vi "gyro.vi"(0 "startspeed":dbl, 1 "left":dbl, 5 "kp- left":dbl, 7 "kp- right":dbl, 9 "kp+ left":dbl, 11 "kp+ right":dbl, 12 "right":dbl) -> ()   [LabVIEW 2016]
uses:
  <vilib>/Rock Robotics/WPI/Utilities/WPI_GetSetVariantRefNum.vi
panel:
  out "angle 2":dbl
  out "pi":dbl
  out "angle":dbl=360.0
  in  "Delay (s)":dbl
  in  "Feed time (s)":dbl=0.05
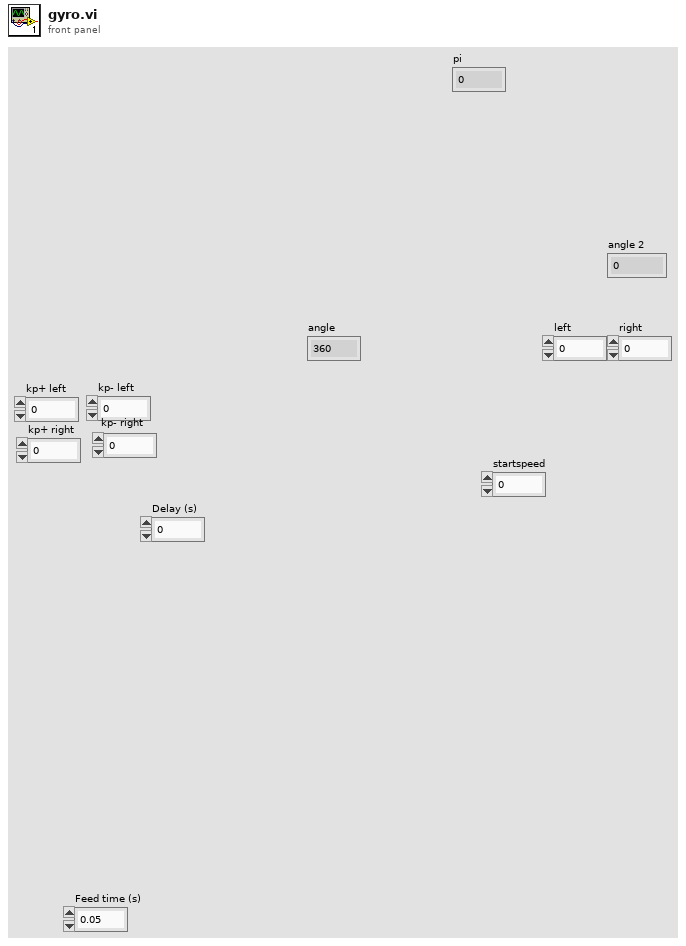
[diagram p1: front panel]
types:
  T1 = typedef "WPI_GyroDevRef.ctl" = cluster{"DevStatus":errorcluster, "Analog Channel":T2, "Offset":dbl, "Gain (VoltsPerDegree/Second)":dbl, "Gyro Type":enum16{"Analog", "XRS450"}, "Handle":i32, "SPI Bus":T3, "Device Found":bool, "Sample Rate":dbl, "Calibrate On Open":bool}
  T2 = typedef "FPGA_AIChannel.ctl" = enum8{"AI 0", "AI 1", "AI 2", "AI 3", "AI MXP 0", "AI MXP 1", "AI MXP 2", "AI MXP 3", "Invalid"}
  T3 = typedef "spi_bus.ctl" = enum16{"SPI On-Board, CS0", "SPI On-Board, CS1", "SPI On-Board, CS2", "SPI On-Board, CS3", "SPI MXP", "Invalid"}
  T4 = typedef "WPI_RobotDriveDevRef.ctl" = cluster{"DevStatus":errorcluster, "Motors[]":T5[], "Square Inputs":bool, "Max Output":dbl}
  T5 = typedef "WPI_MotorControlDeviceRef.ctl" = cluster{"DeviceStatus":errorcluster, "Type":T6, "PWM":cluster{"PWM Channel":T7, "DeadBand":T8}, "CAN":cluster{"Device Number":u8, "SetOutput VI Ref":variant, "GetOutput VI Ref":variant, "Enable VI Ref":variant, "Disable VI Ref":variant, "Data":variant}, "Invert":bool}
  T6 = typedef "WPI_MotorControlType.ctl" = enum16{"PWM", "CAN"}
  T7 = typedef "FPGA_DIOPWMChannel.ctl" = enum8{"PWM 0", "PWM 1", "PWM 2", "PWM 3", "PWM 4", "PWM 5", "PWM 6", "PWM 7", "PWM 8", "PWM 9", "PWM MXP 0", "PWM MXP 1", "PWM MXP 2", "PWM MXP 3", "PWM MXP 4", "PWM MXP 5", "PWM MXP 6", "PWM MXP 7", "PWM MXP 8", "PWM MXP 9", "Invalid"}
  T8 = typedef "WPI_PWMDeadband.ctl" = cluster{"Name":string, "maxPositivePwm":i32, "minPositivePwm":i32, "centerPwm":i32, "maxNegativePwm":i32, "minNegativePwm":i32, "angularRange":u16}
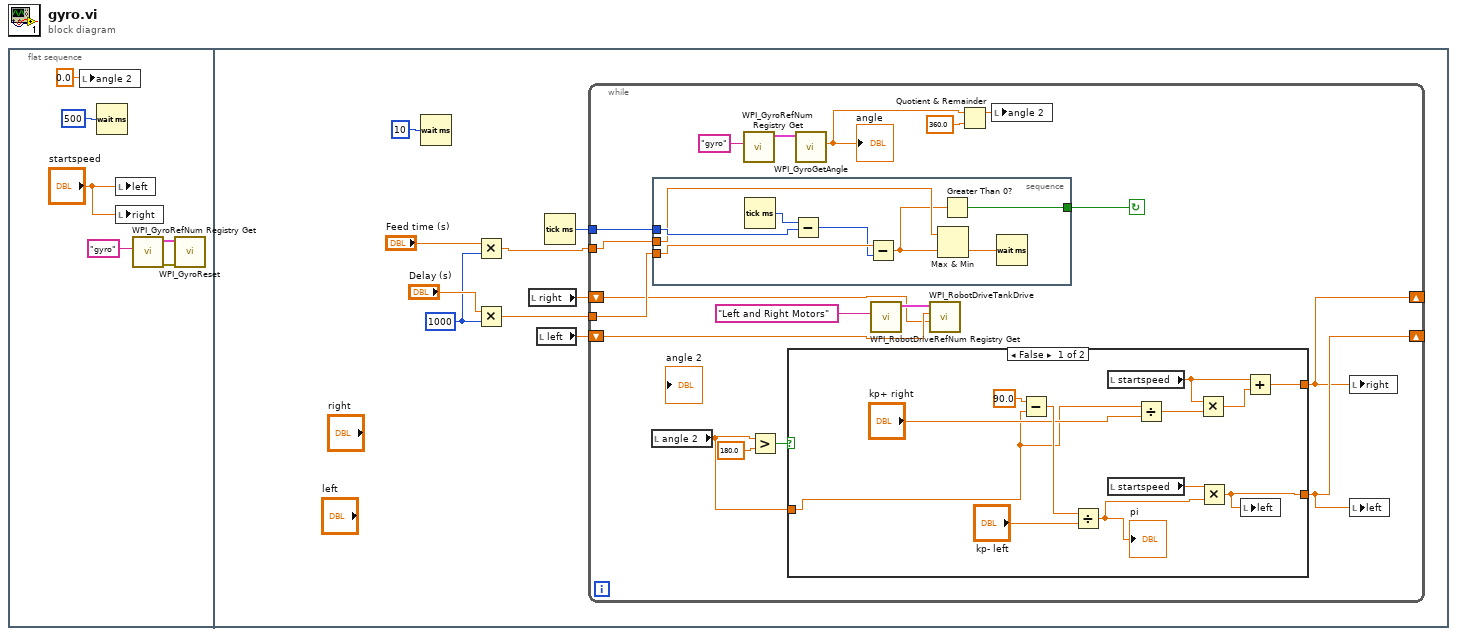
[diagram p0: block diagram]
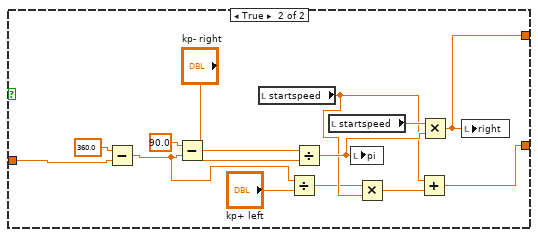
[diagram p2: hidden frame]
diagram:
  n1 = flat-sequence {
    frame #0 {
      n2 = local write "angle 2"(0.0 ("angle")) -> ()
      n3 = Wait (ms)(milliseconds to wait=u32 500) -> ()  [unwired: 1 out]
      n4 = local write "left"("startspeed") -> ()
      n5 = local write "right"("startspeed") -> ()
      n6 = call <vilib>:"WPI_GyroRefNum Registry Get.vi"("refnum name"="gyro") -> ("error out"=w4:errorcluster, "GyroDevRef"=w5:T1)  [unwired: 9 in]
      n7 = call <vilib>:"WPI_GyroReset.vi"("error in"=w4, "GyroDevRef"=w5) -> ()  [unwired: 8 in, 2 out]
    }
    frame #1 {
      w13 = 1000
      n8 = Wait (ms)(milliseconds to wait=u32 10) -> ()  [unwired: 1 out]
      n9 = Multiply(x="Feed time (s)", y=w13) -> (x*y=w12:dbl)
      n10 = Multiply(x="Delay (s)", y=w13) -> (x*y=w11:dbl)
      n11 = local read "right"() -> (w8:dbl)
      n12 = local read "left"() -> (w9:dbl)
      n13 = Tick Count (ms)() -> (millisecond timer value=w10:u32)
      n14 = while {
        tunnel: w11 -> [w31]
        tunnel: w12 -> [w32]
        tunnel: w10 -> [w33]
        shift-right: [w16] -> _
        shift-left: w8 -> [w22]
        shift-right: [w17] -> _
        shift-left: w9 -> [w23]
        stop <- w30 continue-if-true
        n15 = local read "angle 2"() -> (w19:dbl)
        n16 = stacked-sequence {
          tunnel: w33 -> [w67]
          tunnel: w32 -> [w66]
          tunnel: w31 -> [w64]
          tunnel: [w60] -> w30
          frame #0 {
            n17 = Tick Count (ms)() -> (millisecond timer value=w62:u32)
            n18 = Subtract(x=w62, y=w67) -> (x-y=w63:u32)
            n19 = Subtract(x=w64, y=w63) -> (x-y=w61:dbl)
            n20 = Max & Min(x=w66, y=w61) -> (min(x,y)=w65:dbl)  [unwired: 1 out]
            n21 = Greater Than 0?(x=w61) -> (x > 0?=w60:bool)
            n22 = Wait (ms)(milliseconds to wait=w65) -> ()  [unwired: 1 out]
          }
        }
        n23 = call <vilib>:"WPI_GyroRefNum Registry Get.vi"("refnum name"="gyro") -> ("GyroDevRef"=w27:T1)  [unwired: 9 in, 1 out]
        n24 = Greater?(x=w19, y=180.0) -> (0:w20:bool)
        n25 = case shown="False" w20 {
          tunnel: w19 -> [w34 w57]
          tunnel: [w42 w56] -> w16
          tunnel: [w44 w53] -> w17
          frame False {
            n26 = Subtract(x=90.0, y=w34) -> (x-y=w37:dbl)
            n27 = Divide(x=w37, y="kp- left") -> (x/y=w39:dbl)
            "pi" <- w39
            n28 = local read "startspeed"() -> (w40:dbl)
            n29 = local read "startspeed"() -> (w45:dbl)
            n30 = Divide(x=w34, y="kp+ right") -> (x/y=w36:dbl)
            n31 = Multiply(x=w40, y=w36) -> (x*y=w41:dbl)
            n32 = Multiply(x=w45, y=w39) -> (x*y=w44:dbl)
            n33 = local write "left"(w44) -> ()
            n34 = Add(x=w40, y=w41) -> (x+y=w42:dbl)
          }
          frame True {
            n35 = Subtract(x=360.0, y=w57) -> (x-y=w46:dbl)
            n36 = Subtract(x=90.0, y=w46) -> (x-y=w50:dbl)
            n37 = local read "startspeed"() -> (w51:dbl)
            n38 = Divide(x=w46, y="kp+ left") -> (x/y=w48:dbl)
            n39 = Divide(x=w50, y="kp- right") -> (x/y=w54:dbl)
            n40 = local read "startspeed"() -> (w59:dbl)
            n41 = local write "pi"(w54) -> ()
            n42 = Multiply(x=w48, y=w51) -> (x*y=w52:dbl)
            n43 = Add(x=w51, y=w52) -> (x+y=w53:dbl)
            n44 = Multiply(x=w59, y=w54) -> (x*y=w56:dbl)
            n45 = local write "right"(w56) -> ()
          }
        }
        n46 = call <vilib>:"WPI_GyroGetAngle.vi"("GyroDevRef"=w27) -> ("Angle"=w18:dbl)  [unwired: 6 in, 4 out]
        "angle" <- w18
        n47 = call <vilib>:"WPI_RobotDriveRefNum Registry Get.vi"("refnum name"="Left and Right Motors") -> ("RobotDriveDevRef"=w29:T4)  [unwired: 1 in, 9 out]
        n48 = call <vilib>:"WPI_RobotDriveTankDrive.vi"("Right axis value"=w22, "Left axis value"=w23, "RobotDriveDevRef"=w29) -> ()  [unwired: 6 in, 3 out]
        n49 = Quotient & Remainder(x=w18, y=360.0) -> (x-y*floor(x/y)=w24:dbl)  [unwired: 1 out]
        n50 = local write "angle 2"(w24) -> ()
        n51 = local write "right"(w16) -> ()
        n52 = local write "left"(w17) -> ()
      }
    }
  }
